vi "CreateNewWizard_Interface.vi"() -> (3 "InterfaceTable":T1)   [LabVIEW 2020, in "Add Actor Interface.lvlib"]
doc: "NI Confidential \n\n/**\n@brief This VI tells the framework which VIs to call when an event happens related to one of your items.\n\n@author Joel Dixon\n\n@par Sample_Item_Interface.vi\n For each of the entries in the InterfaceTable, pass in a string representing a relative path to a VI which implements that method. Methods include Init, Exit, OnCommand, OnDropFiles, and OnSelect. \n\n@param \"InterfaceTable\" [out] \nThis is an array of strings passed back to the framework so it knows which VIs should be called under what circumstances.\n*/"
uses:
  Add Actor Interface.lvlib
  <resource>/Framework/Providers/API/CreateNewWizard_Interface.ctl
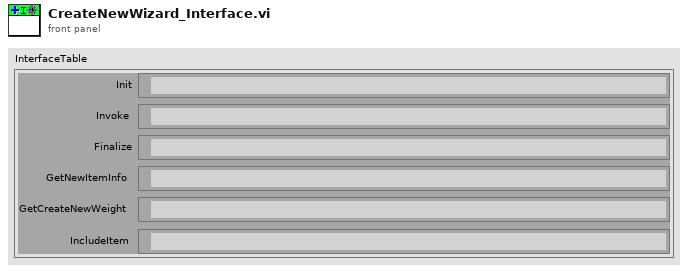
[diagram p1: front panel]
types:
  T1 = typedef "CreateNewWizard_Interface.ctl" = cluster{"Init":path, "Invoke":path, "Finalize":path, "GetNewItemInfo":path, "GetCreateNewWeight":path, "IncludeItem":path}
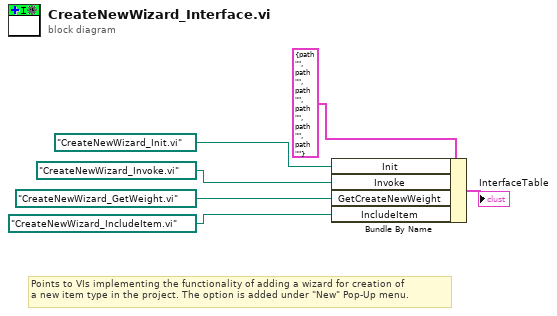
[diagram p0: block diagram]
diagram:
  # "Points to VIs implementing the functionality of adding a wizard for creation of \na new item type in the project. The option is added under \"New\" Pop-Up menu."
  n1 = Bundle By Name(cluster=T1 {"Init"=path "", "Invoke"=path "", "Finalize"=path "", "GetNewItemInfo"=path "", "GetCreateNewWeight"=path "", "IncludeItem"=path ""} ("InterfaceTable"), "Init"=path "CreateNewWizard_Init.vi" ("vi path"), "Invoke"=path "CreateNewWizard_Invoke.vi" ("vi path"), "GetCreateNewWeight"=path "CreateNewWizard_GetWeight.vi", "IncludeItem"=path "CreateNewWizard_IncludeItem.vi") -> (→"InterfaceTable":T1)
